vi "PFI-28000-System_Daemon.vi"(0 "PFI-28000-System":refnum<class "PFI-28000-System.lvclass">) -> ()   [LabVIEW 2017, in "PFI-28000-System.lvclass"]
uses:
  PFI-28000-System.lvclass
  C:/wc/07143 Precision Filters 28000 Support/Driver/source/Base/PFI-28000-Base.lvclass
  Utilities/PFI-28000-Utils.lvlib
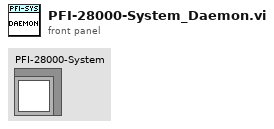
[diagram p1: front panel]
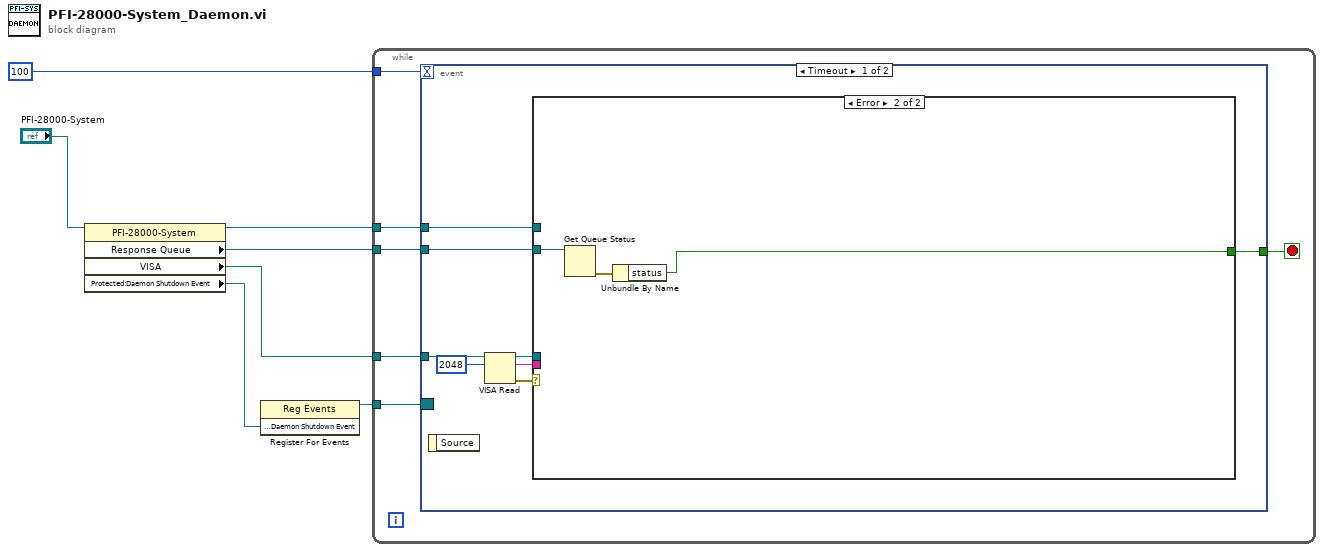
[diagram p0: block diagram]
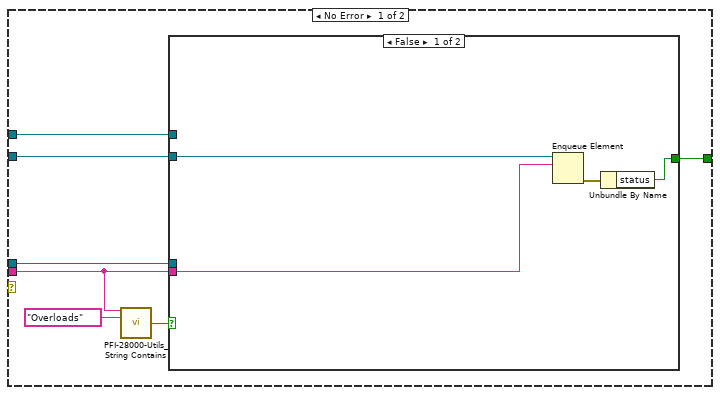
[diagram p2: hidden frame]
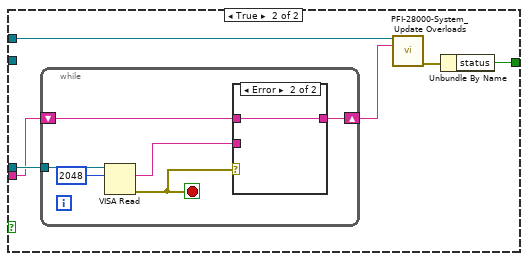
[diagram p3: hidden frame]
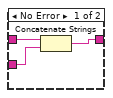
[diagram p4: hidden frame]
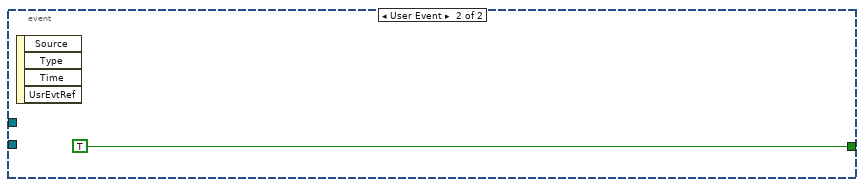
[diagram p5: hidden frame]
diagram:
  n1 = property class="PFI-28000-System"(reference="PFI-28000-System") -> (reference out=w1:refnum<class "PFI-28000-System.lvclass">, "Response Queue"=w4:refnum<queue>, "VISA"=w3:refnum<visa-resource-name>, "Protected:Daemon Shutdown Event"=w2:refnum<user-event>)  [unwired: 1 in, 1 out]
  n2 = register-events(w2) -> (reference out=w7:refnum<event-registration>)  [unwired: 2 in, 1 out]
  n3 = while {
    tunnel: w7 -> [w13]
    tunnel: w3 -> [w11]
    tunnel: w4 -> [w10]
    tunnel: 100 -> [w9]
    tunnel: w1 -> [w8]
    stop <- w12 stop-if-true
    n4 = event shown="[0] Timeout" {
      selector: w13 -> [_ _]
      dyn-events: _ -> [_ _]
      timeout: w9 -> [_ _]
      tunnel: [w15 TRUE] -> w12
      tunnel: w11 -> [w20 _]
      tunnel: w10 -> [w16 _]
      tunnel: w8 -> [w14 _]
      event Timeout {
        n5 = event-data() -> ()  [unwired: 1 in, 1 out]
        n6 = VISA Read(VISA resource name=w20, byte count=u32 2048) -> (VISA resource name out=w17:refnum<visa-resource-name>, read buffer=w18:string, error out=w19:errorcluster)  [unwired: 1 in, 1 out]
        n7 = case shown="Error" w19 {
          tunnel: w18 -> [w24 _]
          tunnel: w17 -> [w28 _]
          tunnel: w16 -> [w27 w51]
          tunnel: [w26 w49] -> w15
          tunnel: w14 -> [w22 _]
          frame No Error {
            n8 = call "PFI-28000-Utils_String Contains.vi"("String"=w24, "Value"="Overloads" ("empty string")) -> ("Contains"=w23:bool)  [unwired: 11 in, 2 out]
            n9 = case shown="False" w23 {
              tunnel: w28 -> [_ w38]
              tunnel: w24 -> [w29 w37]
              tunnel: w27 -> [w32 _]
              tunnel: [w30 w36] -> w26
              tunnel: w22 -> [_ w35]
              frame False {
                n10 = Enqueue Element(queue=w32, element=w29) -> (error out=w31:errorcluster)  [unwired: 2 in, 2 out]
                n11 = Unbundle By Name(w31) -> ("status"=w30:bool)
              }
              frame True {
                n12 = while {
                  tunnel: w38 -> [w44]
                  shift-right: [w41] -> w33
                  shift-left: w37 -> [w42]
                  stop <- w39 stop-if-true
                  n13 = VISA Read(VISA resource name=w44, byte count=u32 2048) -> (read buffer=w40:string, error out=w39:errorcluster)  [unwired: 1 in, 2 out]
                  n14 = case shown="Error" w39 {
                    tunnel: w42 -> [w47 w48]
                    tunnel: [w46 w48] -> w41
                    tunnel: w40 -> [w45 _]
                    frame No Error {
                      n15 = Concatenate Strings(w47, w45) -> (w46:string)
                    }
                    frame Error {
                    }
                  }
                }
                n16 = call "PFI-28000-System_Update Overloads.vi"("PFI-28000-System in"=w35, "String"=w33) -> ("error out"=w34:errorcluster)  [unwired: 12 in, 1 out]
                n17 = Unbundle By Name(w34) -> ("status"=w36:bool)
              }
            }
          }
          frame Error {
            n18 = Get Queue Status(queue=w51) -> (error out=w50:errorcluster)  [unwired: 2 in, 7 out]
            n19 = Unbundle By Name(w50) -> ("status"=w49:bool)
          }
        }
      }
      event User Event {
        n20 = event-data() -> ()  [unwired: 1 in, 4 out]
      }
    }
  }
